vi "unpack_controls.vi"   [LabVIEW 2015]
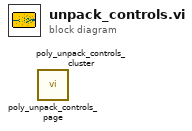
[diagram p0: block diagram]
diagram:
  n1 = call "poly_unpack_controls_page.vi"() -> ()  [unwired: 15 in, 1 out]
  n2 = call "poly_unpack_controls_cluster.vi"() -> ()  [unwired: 15 in, 1 out]
